vi "slope2angle.vi"(11 "slope array":dbl[](array[numeric])) -> (3 "x/y":dbl[](array[numeric]))   [LabVIEW 2017]
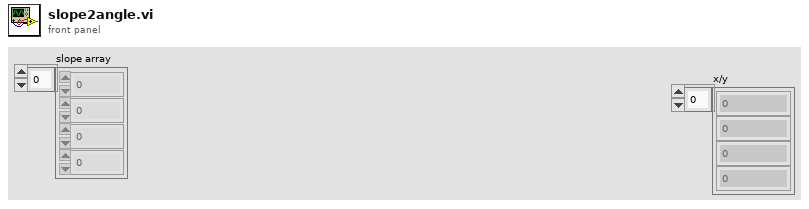
[diagram p1: front panel]
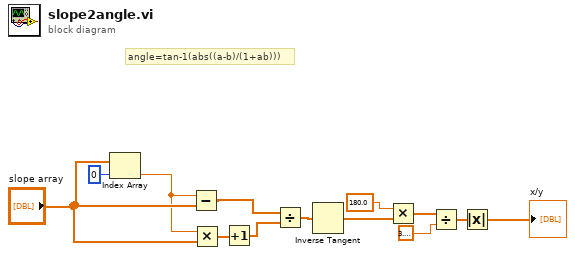
[diagram p0: block diagram]
diagram:
  # "angle=tan-1(abs((a-b)/(1+ab)))"
  n1 = Index Array(array="slope array", index=0) -> (element=w4:dbl)
  n2 = Subtract(x=w4, y="slope array") -> (x-y=w3:dbl[])
  n3 = Multiply(x=w4, y="slope array") -> (x*y=w11:dbl[])
  n4 = Increment(x=w11) -> (x+1=w10:dbl[])
  n5 = Divide(x=w3, y=w10) -> (x/y=w9:dbl[])
  n6 = Inverse Tangent(1:w9) -> (0:w6:dbl[])
  n7 = Multiply(x=180.0, y=w6) -> (x*y=w5:dbl[])
  n8 = Divide(x=w5, y=3.141592653589793) -> (x/y=w2:dbl[])
  n9 = Absolute Value(x=w2) -> (abs(x)=→"x/y":dbl[])
